vi "Bckup_Dcode.vi"(8 "error in (no error)":errorcluster, 10 "Table Name":string, 11 "Refnum in":T1) -> (0 "error out":errorcluster, 2 "DCode":string[](array[string]), 3 "Refnum out":T1)   [LabVIEW 2020]
uses:
  <vilib>/addons/database/Connection.llb/Conn ObjectReference.ctl
  <vilib>/addons/database/Connection.llb/Conn Execute.vi
  <vilib>/addons/database/Recordset.llb/Rec Fetch Recordset Data (R).vi
  <vilib>/addons/database/Recordset.llb/Rec Destroy - Connection.vi
  <vilib>/addons/database/NI_Database_API.lvlib
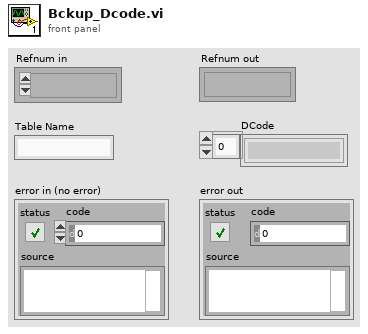
[diagram p1: front panel]
types:
  T1 = typedef "NI_Database_API.lvlib/Conn ObjectReference.ctl" = refnum<k1>
  T2 = typedef "NI_Database_API.lvlib/Rec ObjectReference.ctl" = refnum<k1>
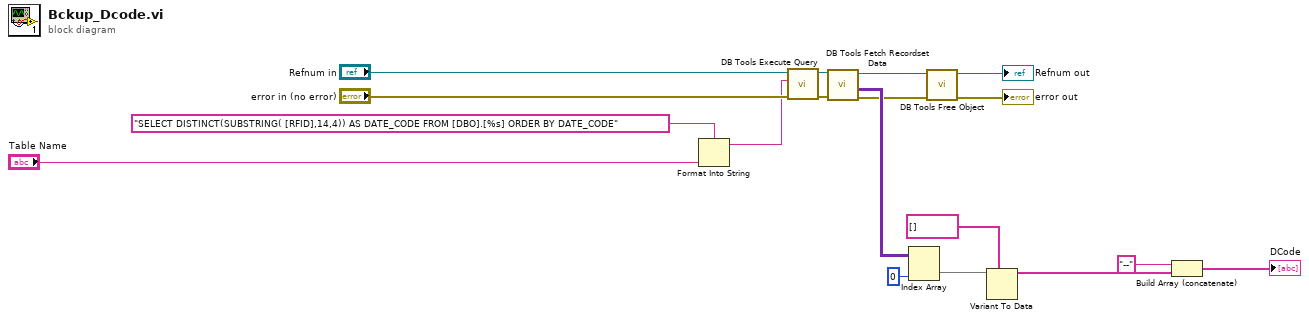
[diagram p0: block diagram]
diagram:
  n1 = Format Into String(format string="SELECT DISTINCT(SUBSTRING( [RFID],14,4)) AS DATE_CODE FROM [DBO].[%s] ORDER BY DATE_CODE" ("userID"), "Table Name") -> (resulting string=w3:string)  [unwired: 2 in, 1 out]
  n2 = call-poly <vilib>:"DB Tools Execute Query.vi"("error in (no error)"="error in (no error)", "SQL query"=w3, "connection reference"="Refnum in") -> ("error out"=w9:errorcluster, "recordset reference"=w8:T2)  [unwired: 5 in]
  n3 = call-poly <vilib>:"DB Tools Fetch Recordset Data.vi"("error in (no error)"=w9, "recordset reference"=w8) -> ("error out"=w6:errorcluster, "recordset data"=w14:variant[][], "recordset reference out"=w7:T2)  [unwired: 3 in]
  n4 = Index Array(array=w14, index (col)=0 ("disabled index (col)")) -> (element=w16:variant[])  [unwired: 1 in]
  n5 = call-poly <vilib>:"DB Tools Free Object.vi"("error in (no error)"=w6, "recordset reference"=w7) -> ("error out"=→"error out":errorcluster, "connection reference"=→"Refnum out":T1)  [unwired: 8 in]
  n6 = Variant To Data(type=string[] [] ("Item Names"), Variant=w16) -> (data=w18:string[])  [unwired: 1 in, 1 out]
  n7 = Build Array (concatenate)("--", w18) -> (→"DCode":string[])
